vi "Dresden Edit Recipe(in).vi"() -> ()   [LabVIEW 2009]
uses:
  <vilib>/Utility/file.llb/Read From Spreadsheet File (string).vi
  kernel32.dll
panel:
  out "OKTO":bool
  out "error out":errorcluster
  out "Data":string[][](array[string])
  in  "R General_tab":enum32{"Page 1", "Page 2"}(tab)
  in  "Cancel":bool
  in  "Thickness_Monitor_Active":bool
  in  "Recipe_selection tab":T1(tab)
  in  "R_Simple_Coating Type Selection":T2(radio)
  in  "R_Single_Coating Type Selection_tab":T3(tab)
  in  "R_Single Microwave Time":dbl caption="sec"
  in  "R_Single Microwave Power":dbl caption="Watt"
  in  "R Single Pass Number":dbl
  in  "R_Single DC_Material ok":bool
  in  "R_Single DC_Mat_sel":u64(ring) items=["Other", "Ag", "AgBr", "AgCl", "Al", "Al2O3", "As", "Au", "B", "Ba", "Be", "Bi", "Bi2O3", "C (Diamond)", "C (Graphite)", "Ca", "CaF", "Cd", "CdS", "CdSe", "CdTe", "CeF3", "CeO", "Cr", "Cr2O3", "Co", "Cu", "Cu2S (A)", "Cu2S (B)", "CuS", "Dy", "Er", "Fe", "Ga", "GaAs", "Gd", "Ge", "Hf", "HfO2", "Hg", "Ho", "In", "InSb", "In2O3", "Ir", "KCl", "La", "LaF3", "LaO3", "Li", "LiF", "Mg", "MgF2", "MgO", "Mn", "MnS", "Mo", "Na", "NaCl", "NdF3", "Nd2O3", "Ni", "Nb", "Nb2O5", "Pb", "PbS", "Pd", "Pt", "Re", "Rh", "Rb", "S", "Sb", "Sc", "Se", "Si", "SiO", "SiO2", "Sm", "Sn", "Ta", "Ta2O5", "Te", "Tb", "ThF4", "Ti", "TiO2", "TiO", "Tl", "U", "V", "W", "WC", "Y", "Y2O3", "Yb", "Zn", "ZnO", "ZnSe", "ZnS", "Zr", "ZrO2", "Si3N4", "ITO", "PbI2"]
  in  "R Single DC Target material":string
  in  "R_DC_Chamber_selection":enum32{"Chamber II", "Chamber III"}(radio)
  in  "Power_singledc_list_open":bool
  in  "R_Single RF Material ok":bool
  in  "R_Single RF_Mat_sel":u64(ring) items=["Other", "Ag", "AgBr", "AgCl", "Al", "Al2O3", "As", "Au", "B", "Ba", "Be", "Bi", "Bi2O3", "C (Diamond)", "C (Graphite)", "Ca", "CaF", "Cd", "CdS", "CdSe", "CdTe", "CeF3", "CeO", "Cr", "Cr2O3", "Co", "Cu", "Cu2S (A)", "Cu2S (B)", "CuS", "Dy", "Er", "Fe", "Ga", "GaAs", "Gd", "Ge", "Hf", "HfO2", "Hg", "Ho", "In", "InSb", "In2O3", "Ir", "KCl", "La", "LaF3", "LaO3", "Li", "LiF", "Mg", "MgF2", "MgO", "Mn", "MnS", "Mo", "Na", "NaCl", "NdF3", "Nd2O3", "Ni", "Nb", "Nb2O5", "Pb", "PbS", "Pd", "Pt", "Re", "Rh", "Rb", "S", "Sb", "Sc", "Se", "Si", "SiO", "SiO2", "Sm", "Sn", "Ta", "Ta2O5", "Te", "Tb", "ThF4", "Ti", "TiO2", "TiO", "Tl", "U", "V", "W", "WC", "Y", "Y2O3", "Yb", "Zn", "ZnO", "ZnSe", "ZnS", "Zr", "ZrO2", "Si3N4", "ITO", "PbI2"]
  in  "R Single RF Target material":string
  in  "R Single RF Ramp down":bool
  in  "R Single RF Ramp down Time":dbl caption="sec"
  in  "R Single RF Ramp up Time":dbl caption="sec"
  in  "R Single RF Ramp up":bool
  in  "Power_single_rf_list_open":bool
  in  "Power_list_open_multi":bool
  in  "R Cmb Ch3 Material ok":bool
  in  "R Cmb Ch3 Mat_sel":u64(ring) items=["Other", "Ag", "AgBr", "AgCl", "Al", "Al2O3", "As", "Au", "B", "Ba", "Be", "Bi", "Bi2O3", "C (Diamond)", "C (Graphite)", "Ca", "CaF", "Cd", "CdS", "CdSe", "CdTe", "CeF3", "CeO", "Cr", "Cr2O3", "Co", "Cu", "Cu2S (A)", "Cu2S (B)", "CuS", "Dy", "Er", "Fe", "Ga", "GaAs", "Gd", "Ge", "Hf", "HfO2", "Hg", "Ho", "In", "InSb", "In2O3", "Ir", "KCl", "La", "LaF3", "LaO3", "Li", "LiF", "Mg", "MgF2", "MgO", "Mn", "MnS", "Mo", "Na", "NaCl", "NdF3", "Nd2O3", "Ni", "Nb", "Nb2O5", "Pb", "PbS", "Pd", "Pt", "Re", "Rh", "Rb", "S", "Sb", "Sc", "Se", "Si", "SiO", "SiO2", "Sm", "Sn", "Ta", "Ta2O5", "Te", "Tb", "ThF4", "Ti", "TiO2", "TiO", "Tl", "U", "V", "W", "WC", "Y", "Y2O3", "Yb", "Zn", "ZnO", "ZnSe", "ZnS", "Zr", "ZrO2", "Si3N4", "ITO", "PbI2"]
  in  "R Cmb Ch3 Target material":string
  in  "R_Cmb Ch2_Material ok":bool
  in  "R_Cmb Ch2_Mat_sel":u64(ring) items=["Other", "Ag", "AgBr", "AgCl", "Al", "Al2O3", "As", "Au", "B", "Ba", "Be", "Bi", "Bi2O3", "C (Diamond)", "C (Graphite)", "Ca", "CaF", "Cd", "CdS", "CdSe", "CdTe", "CeF3", "CeO", "Cr", "Cr2O3", "Co", "Cu", "Cu2S (A)", "Cu2S (B)", "CuS", "Dy", "Er", "Fe", "Ga", "GaAs", "Gd", "Ge", "Hf", "HfO2", "Hg", "Ho", "In", "InSb", "In2O3", "Ir", "KCl", "La", "LaF3", "LaO3", "Li", "LiF", "Mg", "MgF2", "MgO", "Mn", "MnS", "Mo", "Na", "NaCl", "NdF3", "Nd2O3", "Ni", "Nb", "Nb2O5", "Pb", "PbS", "Pd", "Pt", "Re", "Rh", "Rb", "S", "Sb", "Sc", "Se", "Si", "SiO", "SiO2", "Sm", "Sn", "Ta", "Ta2O5", "Te", "Tb", "ThF4", "Ti", "TiO2", "TiO", "Tl", "U", "V", "W", "WC", "Y", "Y2O3", "Yb", "Zn", "ZnO", "ZnSe", "ZnS", "Zr", "ZrO2", "Si3N4", "ITO", "PbI2"]
  in  "R Cmb Ch2 Target material":string
  in  "R Cmb Number of cycle":dbl
  in  "R_First_stop_selection":enum32{"Chamber II", "Chamber III"}(radio)=enum."Chamber III"
  in  "R_Cmb_Ch2_Web_speed":dbl
  in  "R_Cmb_Ch3_Web_speed":dbl
  in  "Substrate Material":string
  in  "Recipe Name":string
  in  "R_Recipe_type_selection":enum32{"Single Recipe", "Combination Sputter"}(radio)
  in  "R_Web_selection":enum32{"Web", "Other"}(radio)=enum."Other"
  in  "Web_selection_tab":T4(tab)
  in  "R Web thickness":dbl
  in  "R Maximum diameter":dbl format="%.1f"
  in  "R Minimum diameter":dbl format="%.1f"
  in  "R Web speed(cm/min)":dbl
  in  "R Tension Value":dbl
  out "R  Total length":dbl caption="cm" format="%.2f"
  in  "Calculate":bool
  in  "R_Thickness Selection":enum32{"Thickness", "Time"}(radio)
  in  "R_Target Thickness Value":dbl format="%.2f"
  in  "R_Duration":dbl caption="%"
  in  "R Set Pressure mtorr":dbl caption="mbar" format="%.1f"
  in  "R Argon Flow sccm":dbl caption="sccm"
  in  "R Z_factor":dbl format="%_3f"
  in  "R Material_density":dbl caption="g/cm3" format="%_3f"
  in  "OK":bool caption="OK2"
  in  "R Toooling_factor":dbl caption="%"
  out "Calculated_total_length_dc":dbl
  out "Lap":dbl
  in  "Diameter":dbl
  in  "Multilayer_power_tab":enum32{"Page 1", "Page 2"}(tab)
  in  "R Cmb Interval length 1":dbl
  in  "R Cmb Ch3 Step1 Coating Power":dbl caption="Watt"
  in  "R Cmb Step1 Coating Power Active":bool
  in  "R Cmb Ch2 Step1 Coating Power":dbl caption="Watt"
  in  "R Cmb Interval length 2":dbl
  in  "R Cmb Ch3 Step2 Coating Power":dbl caption="Watt"
  in  "R Cmb Step2 Coating Power Active":bool
  in  "R Cmb Ch2 Step2 Coating Power":dbl caption="Watt"
  in  "R Cmb Interval length 3":dbl
  in  "R Cmb Ch3 Step3 Coating Power":dbl caption="Watt"
  in  "R Cmb Step3 Coating Power Active":bool
  in  "R Cmb Ch2 Step3 Coating Power":dbl caption="Watt"
  in  "R Cmb Interval length 4":dbl
  in  "R Cmb Ch3 Step4 Coating Power":dbl caption="Watt"
  in  "R Cmb Step4 Coating Power Active":bool
  in  "R Cmb Ch2 Step4 Coating Power":dbl caption="Watt"
  in  "R Cmb Interval length 5":dbl
  in  "R Cmb Ch3 Step5 Coating Power":dbl caption="Watt"
  in  "R Cmb Step5 Coating Power Active":bool
  in  "R Cmb Ch2 Step5 Coating Power":dbl caption="Watt"
  in  "R Cmb Interval length 6":dbl
  in  "R Cmb Ch3 Step6 Coating Power":dbl caption="Watt"
  in  "R Cmb Step6 Coating Power Active":bool
  in  "R Cmb Ch2 Step6 Coating Power":dbl caption="Watt"
  in  "R Cmb Interval length 7":dbl
  in  "R Cmb Ch3 Step7 Coating Power":dbl caption="Watt"
  in  "R Cmb Step7 Coating Power Active":bool
  in  "R Cmb Ch2 Step7 Coating Power":dbl caption="Watt"
  in  "R Cmb Interval length 8":dbl
  in  "R Cmb Ch3 Step8 Coating Power":dbl caption="Watt"
  in  "R Cmb Step8 Coating Power Active":bool
  in  "R Cmb Ch2 Step8 Coating Power":dbl caption="Watt"
  in  "R Cmb Interval length 9":dbl
  in  "R Cmb Ch3 Step9 Coating Power":dbl caption="Watt"
  in  "R Cmb Step9 Coating Power Active":bool
  in  "R Cmb Ch2 Step9 Coating Power":dbl caption="Watt"
  in  "R Cmb Interval length 10":dbl
  in  "R Cmb Ch3 Step10 Coating Power":dbl caption="Watt"
  in  "R Cmb Step10 Coating Power Active":bool
  in  "R Cmb Ch2 Step10 Coating Power":dbl caption="Watt"
  in  "Single_DC_power_power_tab":enum32{"Page 1", "Page 2"}(tab)
  in  "R Single DC Interval length1":dbl
  in  "R Single DC Step1 Coating Power Active":bool
  in  "R Single DC Step1 Coating Power":dbl caption="Watt"
  in  "R Single DC Interval length2":dbl
  in  "R Single DC Step2 Coating Power Active":bool
  in  "R Single DC Step2 Coating Power":dbl caption="Watt"
  in  "R Single DC Step3 Coating Power Active":bool
  in  "R Single DC Step3 Coating Power":dbl caption="Watt"
  in  "R Single DC Interval length3":dbl
  in  "R Single DC Step4 Coating Power Active":bool
  in  "R Single DC Step4 Coating Power":dbl caption="Watt"
  in  "R Single DC Interval length4":dbl
  in  "R Single DC Step5 Coating Power Active":bool
  in  "R Single DC Step5 Coating Power":dbl caption="Watt"
  in  "R Single DC Interval length5":dbl
  in  "R Single DC Step6 Coating Power Active":bool
  in  "R Single DC Step6 Coating Power":dbl caption="Watt"
  in  "R Single DC Interval length6":dbl
  in  "R Single DC Step7 Coating Power Active":bool
  in  "R Single DC Step7 Coating Power":dbl caption="Watt"
  in  "R Single DC Interval length7":dbl
  in  "R Single DC Step8 Coating Power Active":bool
  in  "R Single DC Step8 Coating Power":dbl caption="Watt"
  in  "R Single DC Interval length8":dbl
  in  "R Single DC Step9 Coating Power Active":bool
  in  "R Single DC Step9 Coating Power":dbl caption="Watt"
  in  "R Single DC Interval length9":dbl
  in  "R Single DC Step10 Coating Power Active":bool
  in  "R Single DC Step10 Coating Power":dbl caption="Watt"
  in  "R Single DC Interval length10":dbl
  in  "Single_RF_power_power_tab":enum32{"Page 1", "Page 2"}(tab)
  in  "R Single RF  Step1 Coating Power":dbl caption="Watt"
  in  "R Single RF Step1 Coating Power Active":bool
  in  "R Single RF Step2 Coating Power":dbl caption="Watt"
  in  "R Single RF Step2 Coating Power Active":bool
  in  "R Single RF Step3 Coating Power":dbl caption="Watt"
  in  "R Single RF Step3 Coating Power Active":bool
  in  "R Single RF Step4 Coating Power":dbl caption="Watt"
  in  "R Single RF Step4 Coating Power Active":bool
  in  "R Single RF Step5 Coating Power":dbl caption="Watt"
  in  "R Single RF Step5 Coating Power Active":bool
  in  "R Single RF Interval length":dbl
  in  "R Single RF Interval length2":dbl
  in  "R Single RF Interval length3":dbl
  in  "R Single RF Interval length4":dbl
  in  "R Single RF Interval length5":dbl
  in  "R Single RF Step6 Coating Power":dbl caption="Watt"
  in  "R Single RF Step6 Coating Power Active":bool
  in  "R Single RF Interval length6":dbl
  in  "R Single RF Step7 Coating Power":dbl caption="Watt"
  in  "R Single RF Step7 Coating Power Active":bool
  in  "R Single RF Interval length7":dbl
  in  "R Single RF Step8 Coating Power":dbl caption="Watt"
  in  "R Single RF Step8 Coating Power Active":bool
  in  "R Single RF Interval length8":dbl
  in  "R Single RF Step9 Coating Power":dbl caption="Watt"
  in  "R Single RF Step9 Coating Power Active":bool
  in  "R Single RF Interval length9":dbl
  in  "R Single RF Step10 Coating Power":dbl caption="Watt"
  in  "R Single RF Step10 Coating Power Active":bool
  in  "R Single RF Interval length10":dbl
  out "Calculated_total_length_rf":dbl
  out "Calculated_total_length_cmb":dbl
  in  "Path":string
  out "Recipe_path":path
  out "Recipe_cancel":bool
  # "Recipe  Selection"
  # "Web  Selection"
  # "Thickness Monitor Parameters"
  # "Pressure Control Parameters"
  # "Material Density       :"
  # "Argon Flow         :"
  # "Z factor                    :"
  # "Set Pressure        :"
  # "Tooling Factor         :"
  # "Single Process  Selection"
  # "Power Value     :"
  # "Watt"
  # "Duration           :"
  # "sec"
  # "Pass Number    :"
  # "DCPS Parameters"
  # "Target material          :"
  # "RFPS Parameters"
  # "Target material          :"
  # "Ramp Up Time           :"
  # "Ramp Down Time      :"
  # "DCPS Parameters"
  # "Chamber II"
  # "Chamber III"
  # "Target material         :"
  # "Target material          :"
  # "Web Speed                :"
  # "cm/sec"
  # "Web Speed               :"
  # "cm/sec"
  # "Number of cycle:"
  # "First Stop :"
  # "Roll  Parameters"
  # "Minimum Diameter     :"
  # "mm"
  # "Web Speed              :"
  # "cm / min"
  # "Tension Value         :"
  # "Maximum Diameter     :"
  # "mm"
  # "N"
  # "Web Thickness            :"
  # "µm"
  # "Total Length           :"
  # "Other Parameters"
  # "Thickness Selection         :"
  # "Target Thickness Value   :"
  # "kA"
  # "min"
  # "Step List"
  # "CH2-Power(Watt)"
  # "CH3-Power(Watt)"
  # "Interval Length(cm)"
  # "Step 1:"
  # "cm"
  # "cm"
  # "Step 2:"
  # "Step 3:"
  # "cm"
  # "Step 4:"
  # "cm"
  # "Step 5:"
  # "cm"
  # "Step 6:"
  # "cm"
  # "cm"
  # "Step 7:"
  # "cm"
  # "Step 8:"
  # "cm"
  # "Step 9:"
  # "Step 10:"
  # "cm"
  # "Step List"
  # "Interval Length(cm)"
  # "Power(Watt)"
  # "cm"
  # "Step 1            :"
  # "Step 2            :"
  # "cm"
  # "Step 3            :"
  # "cm"
  # "Step 4            :"
  # "cm"
  # "Step 5            :"
  # "cm"
  # "Step 6            :"
  # "cm"
  # "Step 7            :"
  # "cm"
  # "Step 8            :"
  # "cm"
  # "cm"
  # "Step 9            :"
  # "cm"
  # "Step 10          :"
  # "Step List"
  # "Interval Length(cm)"
  # "Power(Watt)"
  # "Step 1    :"
  # "cm"
  # "Step 2    :"
  # "cm"
  # "Step 3    :"
  # "cm"
  # "Step 4    :"
  # "cm"
  # "Step 5    :"
  # "cm"
  # "Step 6    :"
  # "cm"
  # "Step 7    :"
  # "cm"
  # "Step 8    :"
  # "cm"
  # "Step 9    :"
  # "cm"
  # "Step 10  :"
  # "cm"
types:
  T1 = enum32{"Single Recipe                                                                         ", "Multilayer Recipe                                                                  "}
  T2 = enum32{"Microwave Plasma", "DC Sputter", "RF Sputter"}
  T3 = enum32{"Microwave                                          ", "DC Sputter                                                 ", "RF Sputter                                       "}
  T4 = enum32{"Web                                                                                    ", "Other                                                                                    "}
  T5 = enum8{"Enabled", "Disabled", "Disabled and Grayed Out"}
  T6 = enum16{"open", "replace", "create", "open or create", "replace or create", "replace or create with confirmation"}
diagram:
  n1 = stacked-sequence {
    tunnel: [_ _ _ _ _ w820] -> w1
    frame #0 {
      n2 = Wait (ms)(milliseconds to wait=u32 200) -> ()  [unwired: 1 out]
    }
    frame #1 {
      n3 = File Dialog(9:"" ("Path"), 11:path "" ("base path")) -> (0:w10:errorcluster, 1:w11:bool, 3:w9:path)  [unwired: 2 in, 4 out]
      "Recipe_cancel" <- w11
      n4 = case shown="True" w11 {
        tunnel: w10 -> [_ w18]
        tunnel: [w15 path ""] -> w7
        tunnel: w9 -> [w15 _]
        tunnel: [errorcluster {"status"=FALSE, "code"=0, "source"=""} ("error out") w17] -> w8
        frame #0 {
        }
        frame #1 {
          n5 = call <vilib>:"Clear Errors.vi"("error in (no error)"=w18) -> ("error out"=w17:errorcluster)  [unwired: 6 in]
        }
      }
      "Recipe_path" <- w7
      n6 = call <vilib>:"Simple Error Handler.vi"("error in (no error)"=w8) -> ()  [unwired: 4 in, 5 out]
    }
    frame #2 {
      n7 = Wait (ms)(milliseconds to wait=u32 200) -> ()  [unwired: 1 out]
    }
    frame #3 {
      n8 = local read "Recipe_cancel"() -> (w20:bool)
      n9 = case shown="False" w20 {
        frame #0 {
          # "Min Diameter\nMax.Diameter\nWeb Thick\nWeb speed\nTension Value\nTotal Length"
          # "Substrate Material\nRecipe Selection\nWeb select"
          # "Recipe Name"
          # "153"
          # "152"
          # "151"
          # "150"
          # "149"
          # "148"
          # "147"
          # "146"
          # "145"
          # "144"
          # "143"
          # "142"
          # "141"
          # "140"
          # "139"
          # "138"
          # "137"
          # "136"
          # "135"
          # "134"
          # "133"
          # "132"
          # "131"
          # "130"
          # "129"
          # "128"
          # "127"
          # "126"
          # "125"
          # "124"
          # "123"
          # "122"
          # "121"
          # "120"
          # "119"
          # "118"
          # "117"
          # "116"
          # "115"
          # "114"
          # "113"
          # "112"
          # "111"
          # "110"
          # "109"
          # "108"
          # "102"
          # "101"
          # "100"
          # "99"
          # "98"
          # "97"
          # "96"
          # "95"
          # "94"
          # "93"
          # "92"
          # "91"
          # "90"
          # "89"
          # "88"
          # "87"
          # "86"
          # "85"
          # "84"
          # "83"
          # "82"
          # "81"
          # "80"
          # "79"
          # "78"
          # "77"
          # "76"
          # "75"
          # "74"
          # "73"
          # "72"
          # "71"
          # "70"
          # "69"
          # "68"
          # "Target Material"
          # "Ar"
          # "target metarial rf"
          n10 = local read "Recipe_path"() -> (w728:path)
          n11 = call-poly <vilib>:"Read From Spreadsheet File.vi"("file path (dialog if empty)"=w728) -> ("all rows"=w523:string[][])  [unwired: 6 in, 4 out]
          n12 = Index Array(array=w523, index (row) #1=1 ("disabled index (row)"), index (col) #1=3 ("disabled index (col)"), index (row) #2=4 ("disabled index (row)"), index (col) #2=2 ("disabled index (col)"), index (row) #3=7 ("disabled index (row)"), index (col) #3=2 ("disabled index (col)"), index (row) #4=9 ("disabled index (row)"), index (col) #4=3 ("disabled index (col)"), index (row) #5=12 ("disabled index (row)"), index (col) #5=2 ("disabled index (col)"), index (row) #6=13 ("disabled index (row)"), index (col) #6=2 ("disabled index (col)"), index (row) #7=14 ("disabled index (row)"), index (col) #7=2 ("disabled index (col)"), index (row) #8=15 ("disabled index (row)"), index (col) #8=2 ("disabled index (col)"), index (row) #9=16 ("disabled index (row)"), index (col) #9=2 ("disabled index (col)"), index (row) #10=17 ("disabled index (row)"), index (col) #10=3 ("disabled index (col)"), index (row) #11=20 ("disabled index (row)"), index (col) #11=2 ("disabled index (col)"), index (row) #12=21 ("disabled index (row)"), index (col) #12=1 ("disabled index (col)"), index (row) #13=22 ("disabled index (row)"), index (col) #13=3 ("disabled index (col)"), index (row) #14=25 ("disabled index (row)"), index (col) #14=1 ("disabled index (col)"), index (row) #15=27 ("disabled index (row)"), index (col) #15=1 ("disabled index (col)"), index (row) #16=28 ("disabled index (row)"), index (col) #16=1 ("disabled index (col)"), index (row) #17=29 ("disabled index (row)"), index (col) #17=3 ("disabled index (col)"), index (row) #18=34 ("disabled index (row)"), index (col) #18=2 ("disabled index (col)"), index (row) #19=35 ("disabled index (row)"), index (col) #19=2 ("disabled index (col)"), index (row) #20=36 ("disabled index (row)"), index (col) #20=3 ("disabled index (col)"), index (row) #21=37 ("disabled index (row)"), index (col) #21=3 ("disabled index (col)"), index (row) #22=38 ("disabled index (row)"), index (col) #22=2 ("disabled index (col)"), index (row) #23=39 ("disabled index (row)"), index (col) #23=3 ("disabled index (col)"), index (row) #24=40 ("disabled index (row)"), index (col) #24=3 ("disabled index (col)"), index (row) #25=41 ("disabled index (row)"), index (col) #25=2 ("disabled index (col)"), index (row) #26=42 ("disabled index (row)"), index (col) #26=3 ("disabled index (col)"), index (row) #27=43 ("disabled index (row)"), index (col) #27=3 ("disabled index (col)"), index (row) #28=44 ("disabled index (row)"), index (col) #28=2 ("disabled index (col)"), index (row) #29=45 ("disabled index (row)"), index (col) #29=3 ("disabled index (col)"), index (row) #30=46 ("disabled index (row)"), index (col) #30=3 ("disabled index (col)"), index (row) #31=47 ("disabled index (row)"), index (col) #31=2 ("disabled index (col)"), index (row) #32=48 ("disabled index (row)"), index (col) #32=3 ("disabled index (col)"), index (row) #33=49 ("disabled index (row)"), index (col) #33=3 ("disabled index (col)"), index (row) #34=50 ("disabled index (row)"), index (col) #34=2 ("disabled index (col)"), index (row) #35=51 ("disabled index (row)"), index (col) #35=3 ("disabled index (col)"), index (row) #36=52 ("disabled index (row)"), index (col) #36=3 ("disabled index (col)"), index (row) #37=53 ("disabled index (row)"), index (col) #37=2 ("disabled index (col)"), index (row) #38=54 ("disabled index (row)"), index (col) #38=3 ("disabled index (col)"), index (row) #39=55 ("disabled index (row)"), index (col) #39=3 ("index (col)"), index (row) #40=56 ("disabled index (row)"), index (col) #40=2 ("index (col)"), index (row) #41=57 ("disabled index (row)"), index (col) #41=3 ("index (col)"), index (row) #42=58 ("disabled index (row)"), index (col) #42=3 ("index (col)"), index (row) #43=59 ("disabled index (row)"), index (col) #43=2 ("index (col)"), index (row) #44=60 ("disabled index (row)"), index (col) #44=3 ("index (col)"), index (row) #45=61 ("disabled index (row)"), index (col) #45=3 ("index (col)"), index (row) #46=62 ("disabled index (row)"), index (col) #46=2 ("index (col)"), index (row) #47=63 ("disabled index (row)"), index (col) #47=3 ("disabled index (row)"), index (row) #48=64 ("disabled index (row)"), index (col) #48=3 ("disabled index (col)"), index (row) #49=65 ("disabled index (row)"), index (col) #49=2 ("index (col)"), index (row) #50=68 ("disabled index (row)"), index (col) #50=2 ("index (col)"), index (row) #51=69 ("disabled index (row)"), index (col) #51=2 ("index (col)"), index (row) #52=70 ("disabled index (row)"), index (col) #52=2 ("index (col)"), index (row) #53=71 ("disabled index (row)"), index (col) #53=3 ("disabled index (col)"), index (row) #54=72 ("disabled index (row)"), index (col) #54=3 ("index (col)"), index (row) #55=73 ("disabled index (row)"), index (col) #55=2 ("index (col)"), index (row) #56=74 ("disabled index (row)"), index (col) #56=3 ("index (col)"), index (row) #57=75 ("disabled index (row)"), index (col) #57=3 ("index (col)"), index (row) #58=76 ("disabled index (row)"), index (col) #58=2 ("index (col)"), index (row) #59=77 ("disabled index (row)"), index (col) #59=3 ("index (col)"), index (row) #60=78 ("disabled index (row)"), index (col) #60=3 ("index (col)"), index (row) #61=79 ("disabled index (row)"), index (col) #61=2 ("index (col)"), index (row) #62=80 ("disabled index (row)"), index (col) #62=3 ("index (col)"), index (row) #63=81 ("disabled index (row)"), index (col) #63=3 ("index (col)"), index (row) #64=82 ("disabled index (row)"), index (col) #64=2 ("index (col)"), index (row) #65=83 ("disabled index (row)"), index (col) #65=3 ("index (col)"), index (row) #66=84 ("disabled index (row)"), index (col) #66=3 ("index (col)"), index (row) #67=85 ("disabled index (row)"), index (col) #67=2 ("index (col)"), index (row) #68=86 ("disabled index (row)"), index (col) #68=3 ("index (col)"), index (row) #69=87 ("disabled index (row)"), index (col) #69=3 ("index (col)"), index (row) #70=88 ("disabled index (row)"), index (col) #70=2 ("index (col)"), index (row) #71=89 ("disabled index (row)"), index (col) #71=3 ("index (col)"), index (row) #72=90 ("disabled index (row)"), index (col) #72=3 ("disabled index (col)"), index (row) #73=91 ("disabled index (row)"), index (col) #73=2 ("index (col)"), index (row) #74=92 ("disabled index (row)"), index (col) #74=3 ("index (col)"), index (row) #75=93 ("disabled index (row)"), index (col) #75=3 ("index (col)"), index (row) #76=94 ("disabled index (row)"), index (col) #76=2 ("index (col)"), index (row) #77=95 ("disabled index (row)"), index (col) #77=3 ("index (col)"), index (row) #78=96 ("disabled index (row)"), index (col) #78=3 ("index (col)"), index (row) #79=97 ("disabled index (row)"), index (col) #79=2 ("index (col)"), index (row) #80=98 ("disabled index (row)"), index (col) #80=3 ("index (col)"), index (row) #81=99 ("disabled index (row)"), index (col) #81=3 ("index (col)"), index (row) #82=100 ("disabled index (row)"), index (col) #82=2 ("index (col)"), index (row) #83=101 ("disabled index (row)"), index (col) #83=2 ("index (col)"), index (row) #84=102 ("disabled index (row)"), index (col) #84=2 ("index (col)"), index (row) #85=108 ("disabled index (row)"), index (col) #85=2 ("index (col)"), index (row) #86=109 ("disabled index (row)"), index (col) #86=2 ("index (col)"), index (row) #87=110 ("disabled index (row)"), index (col) #87=2 ("index (col)"), index (row) #88=111 ("index (row)"), index (col) #88=2 ("disabled index (col)"), index (row) #89=112 ("index (row)"), index (col) #89=2 ("disabled index (col)"), index (row) #90=113 ("index (row)"), index (col) #90=3 ("disabled index (col)"), index (row) #91=114 ("index (row)"), index (col) #91=3 ("disabled index (col)"), index (row) #92=115 ("index (row)"), index (col) #92=2 ("disabled index (col)"), index (row) #93=116 ("index (row)"), index (col) #93=3 ("disabled index (col)"), index (row) #94=117 ("index (row)"), index (col) #94=3 ("disabled index (col)"), index (row) #95=118 ("index (row)"), index (col) #95=3 ("disabled index (col)"), index (row) #96=119 ("index (row)"), index (col) #96=2 ("disabled index (col)"), index (row) #97=120 ("index (row)"), index (col) #97=3 ("disabled index (col)"), index (row) #98=121 ("index (row)"), index (col) #98=3 ("disabled index (col)"), index (row) #99=122 ("index (row)"), index (col) #99=3 ("disabled index (col)"), index (row) #100=123 ("index (row)"), index (col) #100=2 ("disabled index (col)"), index (row) #101=124 ("index (row)"), index (col) #101=3 ("disabled index (col)"), index (row) #102=125 ("index (row)"), index (col) #102=3 ("disabled index (col)"), index (row) #103=126 ("index (row)"), index (col) #103=3 ("disabled index (col)"), index (row) #104=127 ("index (row)"), index (col) #104=2 ("disabled index (col)"), index (row) #105=128 ("index (row)"), index (col) #105=3 ("disabled index (col)"), index (row) #106=129 ("index (row)"), index (col) #106=3 ("disabled index (col)"), index (row) #107=130 ("index (row)"), index (col) #107=3 ("disabled index (col)"), index (row) #108=131 ("index (row)"), index (col) #108=2 ("disabled index (col)"), index (row) #109=132 ("index (row)"), index (col) #109=3 ("disabled index (col)"), index (row) #110=133 ("index (row)"), index (col) #110=3 ("disabled index (col)"), index (row) #111=134 ("index (row)"), index (col) #111=3 ("disabled index (col)"), index (row) #112=135 ("index (row)"), index (col) #112=2 ("disabled index (col)"), index (row) #113=136 ("index (row)"), index (col) #113=3 ("disabled index (col)"), index (row) #114=137 ("index (row)"), index (col) #114=3 ("disabled index (col)"), index (row) #115=138 ("index (row)"), index (col) #115=3 ("disabled index (col)"), index (row) #116=139 ("index (row)"), index (col) #116=2 ("disabled index (col)"), index (row) #117=140 ("index (row)"), index (col) #117=3 ("disabled index (col)"), index (row) #118=141 ("index (row)"), index (col) #118=3 ("disabled index (col)"), index (row) #119=142 ("index (row)"), index (col) #119=3 ("disabled index (col)"), index (row) #120=143 ("index (row)"), index (col) #120=2 ("disabled index (col)"), index (row) #121=144 ("index (row)"), index (col) #121=3 ("disabled index (col)"), index (row) #122=145 ("index (row)"), index (col) #122=3 ("disabled index (col)"), index (row) #123=146 ("index (row)"), index (col) #123=3 ("disabled index (col)"), index (row) #124=147 ("index (row)"), index (col) #124=2 ("disabled index (col)"), index (row) #125=148 ("index (row)"), index (col) #125=3 ("disabled index (col)"), index (row) #126=149 ("index (row)"), index (col) #126=3 ("disabled index (col)"), index (row) #127=150 ("index (row)"), index (col) #127=3 ("disabled index (col)"), index (row) #128=151 ("index (row)"), index (col) #128=2 ("disabled index (col)"), index (row) #129=152 ("index (row)"), index (col) #129=2 ("disabled index (col)"), index (row) #130=153 ("index (row)"), index (col) #130=2 ("disabled index (col)"), index (row) #131=157 ("index (row)"), index (col) #131=2 ("disabled index (col)"), index (row) #132=158 ("index (row)"), index (col) #132=2 ("disabled index (col)"), index (row) #133=162 ("index (row)"), index (col) #133=2 ("disabled index (col)"), index (row) #134=163 ("index (row)"), index (col) #134=1 ("disabled index (col)"), index (row) #135=164 ("index (row)"), index (col) #135=3 ("disabled index (col)"), index (row) #136=165 ("disabled index (row)"), index (col) #136=2 ("index (col)")) -> (element #1=w437:string, element #2=w436:string, element #3=w502:string, element #4=w519:string, element #5=w518:string, element #6=w517:string, element #7=w516:string, element #8=w515:string, element #9=w514:string, element #10=w513:string, element #11=w512:string, element #12=w24:string, element #13=w276:string, element #14=w511:string, element #15=w275:string, element #16=w274:string, element #17=w273:string, element #18=w272:string, element #19=w270:string, element #20=w21:string, element #21=w268:string, element #22=w22:string, element #23=w267:string, element #24=w266:string, element #25=w265:string, element #26=w263:string, element #27=w262:string, element #28=w261:string, element #29=w260:string, element #30=w259:string, element #31=w258:string, element #32=w257:string, element #33=w256:string, element #34=w255:string, element #35=w253:string, element #36=w252:string, element #37=w251:string, element #38=w130:string, element #39=w129:string, element #40=w128:string, element #41=w127:string, element #42=w126:string, element #43=w125:string, element #44=w124:string, element #45=w123:string, element #46=w122:string, element #47=w121:string, element #48=w120:string, element #49=w119:string, element #50=w118:string, element #51=w117:string, element #52=w116:string, element #53=w115:string, element #54=w114:string, element #55=w113:string, element #56=w112:string, element #57=w111:string, element #58=w110:string, element #59=w109:string, element #60=w108:string, element #61=w107:string, element #62=w106:string, element #63=w105:string, element #64=w104:string, element #65=w103:string, element #66=w102:string, element #67=w101:string, element #68=w100:string, element #69=w99:string, element #70=w98:string, element #71=w97:string, element #72=w96:string, element #73=w95:string, element #74=w94:string, element #75=w93:string, element #76=w92:string, element #77=w91:string, element #78=w90:string, element #79=w89:string, element #80=w88:string, element #81=w87:string, element #82=w86:string, element #83=w85:string, element #84=w29:string, element #85=w23:string, element #86=w84:string, element #87=w83:string, element #88=w82:string, element #89=w28:string, element #90=w81:string, element #91=w80:string, element #92=w78:string, element #93=w77:string, element #94=w76:string, element #95=w75:string, element #96=w74:string, element #97=w73:string, element #98=w72:string, element #99=w71:string, element #100=w70:string, element #101=w69:string, element #102=w68:string, element #103=w67:string, element #104=w66:string, element #105=w65:string, element #106=w64:string, element #107=w63:string, element #108=w62:string, element #109=w61:string, element #110=w60:string, element #111=w59:string, element #112=w58:string, element #113=w57:string, element #114=w56:string, element #115=w55:string, element #116=w54:string, element #117=w53:string, element #118=w52:string, element #119=w51:string, element #120=w50:string, element #121=w49:string, element #122=w48:string, element #123=w47:string, element #124=w46:string, element #125=w45:string, element #126=w44:string, element #127=w43:string, element #128=w42:string, element #129=w41:string, element #130=w40:string, element #131=w39:string, element #132=w38:string, element #133=w37:string, element #134=w36:string, element #135=w35:string, element #136=w34:string)
          n13 = Equal?(x="Chamber III", y=w41) -> (x = y?=w242:bool)
          n14 = Equal?(x="Chamber II", y=w41) -> (x = y?=w243:bool)
          n15 = Build Array(FALSE, w243, w242) -> (w247:bool[])
          n16 = Boolean Array To Number(Boolean array=w247) -> (number=w246:u32)
          n17 = Equal?(x="Active", y=w37) -> (x = y?=w131:bool)
          n18 = Mantissa & Exponent(0:w246) -> (2:w241:dbl)  [unwired: 1 out]
          n19 = Equal?(x="Active", y=w28) -> (x = y?=w611:bool)
          n20 = Equal?(x="Active", y=w77) -> (x = y?=w429:bool)
          n21 = Equal?(x="Active", y=w65) -> (x = y?=w405:bool)
          n22 = Equal?(x="Active", y=w73) -> (x = y?=w421:bool)
          n23 = Equal?(x="Active", y=w69) -> (x = y?=w413:bool)
          n24 = local write "Recipe Name"(w437) -> ()
          n25 = Equal?(x="Active", y=w57) -> (x = y?=w135:bool)
          n26 = Equal?(x="Active", y=w61) -> (x = y?=w136:bool)
          n27 = Scan Value(string=w39, format string="") -> (value=w238:dbl)  [unwired: 1 in, 1 out]
          n28 = case shown="True" w611 {
            frame #0 {
              n29 = local write "R Cmb Step1 Coating Power Active"(TRUE ("R Cmb Step1 Coating Power Active")) -> ()
            }
            frame #1 {
              n30 = local write "R Cmb Step1 Coating Power Active"(TRUE ("R Cmb Step1 Coating Power Active")) -> ()
            }
          }
          n31 = local write "Substrate Material"(w436) -> ()
